vi "Turret Angle.vi"() -> ()   [LabVIEW 2019]
panel:
  in  "Target Angle":dbl
  in  "Turret Angle":dbl
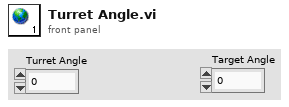
[diagram p1: front panel]
diagram:
